vi "AnalogCNTL_MKSorg.vi"() -> ()   [LabVIEW 2015]
uses:
  <userlib>/caLab/Private/Get_PV-1D.vi
panel:
  in  "LocalEpics":u16(ring) items=["LOCAL", "EPCIS"]
  out "APX:HPC100":dbl
  out "APX:HPC01":dbl
  out "Gain":dbl format="%#_6f"
  out "Vin":dbl
  in  "Vref":dbl min=0.0 max=5.0 step=0.01
  in  "ManualAuto":u16(ring) items=["MANUAL", "AUTO"]
  in  "MFC0:Pcell_RQ":dbl
  out "MFC0:Pcell":dbl
  in  "APX:MFC0_Vin":dbl(knob) min=0.0 max=5.0 step=0.001 scale=0.0..5.0
  in  "stop":bool
  # "MFC0"
  # "OPEN"
  # "CLOSE"
  # "MFC"
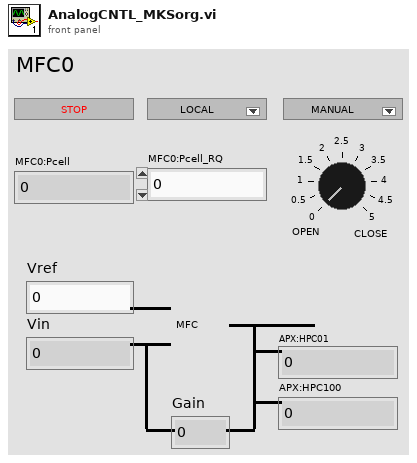
[diagram p1: front panel]
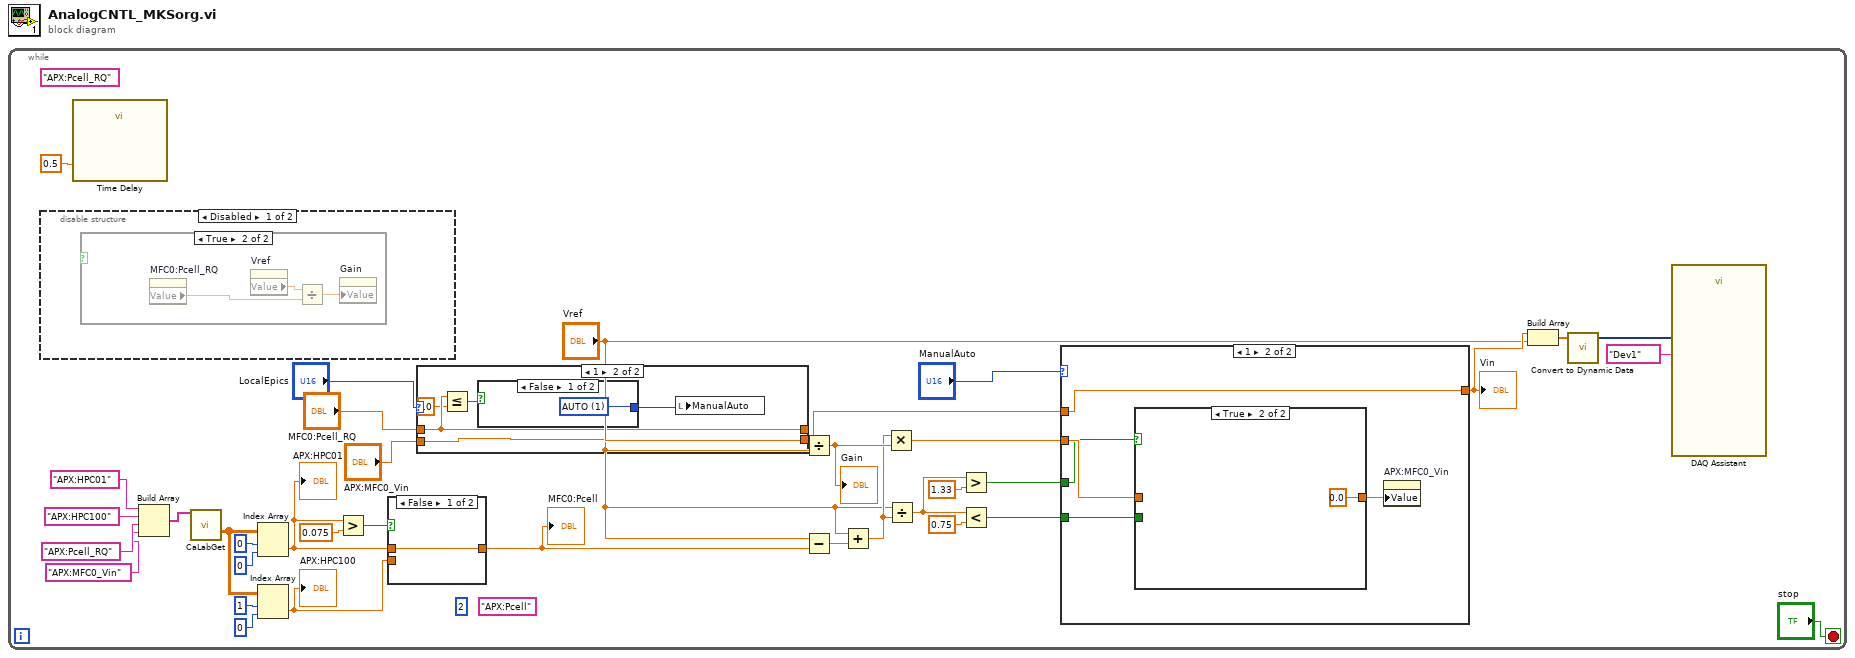
[diagram p0: block diagram]
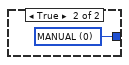
[diagram p4: hidden frame]
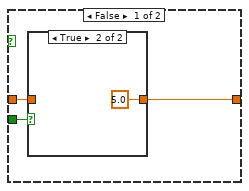
[diagram p8: hidden frame]
diagram:
  n1 = while {
    stop <- "stop" stop-if-true
    (unwired) "APX:Pcell"
    (unwired) "APX:Pcell_RQ"
    (unwired) u16 2 ("y")
    n2 = disable-structure shown="Disabled" {
      frame Disabled {
        n3 = case shown="True" {
          selector: _ -> [_ _]
          frame False {
          }
          frame True {
            n4 = property on="MFC0:Pcell_RQ" class="DigNum (strict)"() -> ("Value"=w49:dbl)  [unwired: 2 in, 2 out]
            n5 = property on="Vref" class="DigNum (strict)"() -> ("Value"=w50:dbl)  [unwired: 2 in, 2 out]
            n6 = Divide(x=w50, y=w49) -> (x/y=w51:dbl)
            n7 = property on="Gain" class="DigNum (strict)"("Value"=w51) -> ()  [unwired: 2 in, 2 out]
          }
        }
      }
      frame Enabled {
      }
    }
    n8 = call "Time Delay"("Delay Time (s)"=0.5) -> ()  [unwired: 10 in, 1 out]
    n9 = Build Array("APX:HPC01", "APX:HPC100", "APX:Pcell_RQ", "APX:MFC0_Vin") -> (w31:string[])
    n10 = call-poly "CaLabGet.vi"("PV Names"=w31) -> ("Value Array (number)"=w27:dbl[][])  [unwired: 8 in, 6 out]
    n11 = Index Array(array=w27, index (row)=0 ("disabled index (col)"), index (col)=0) -> (element=w8:dbl)
    "APX:HPC01" <- w8
    n12 = Index Array(array=w27, index (row)=1 ("disabled index (col)"), index (col)=0) -> (element=w10:dbl)
    "APX:HPC100" <- w10
    n13 = Greater?(x=w8, y=0.075) -> (0:w12:bool)
    n14 = case shown="False" w12 {
      tunnel: w10 -> [_ w39]
      tunnel: [w38 w39] -> w9
      tunnel: w8 -> [w38 _]
      frame False {
      }
      frame True {
      }
    }
    "MFC0:Pcell" <- w9
    n15 = case shown="1" "LocalEpics" {
      tunnel: "MFC0:Pcell_RQ" -> [w41 w45]
      tunnel: [w41 w45] -> w5
      tunnel: [w40 w46] -> w4
      tunnel: "APX:MFC0_Vin" -> [w40 w46]
      frame 0, Default {
      }
      frame 1 {
        n16 = Less Or Equal?(x=w45, y=0.0) -> (x <= y?=w43:bool)
        n17 = case shown="False" w43 {
          tunnel: [w47 w48] -> w42
          frame False {
            w47 = u16 1 items=["MANUAL", "AUTO"] ("ManualAuto")
          }
          frame True {
            w48 = u16 0 items=["MANUAL", "AUTO"] ("ManualAuto")
          }
        }
        n18 = local write "ManualAuto"(w42) -> ()
      }
    }
    n19 = Divide(x="Vref", y=w5) -> (x/y=w16:dbl)
    "Gain" <- w16
    n20 = Subtract(x=w5, y=w9) -> (x-y=w14:dbl)
    n21 = Add(x=w5, y=w14) -> (x+y=w13:dbl)
    n22 = Multiply(x=w13, y=w16) -> (x*y=w34:dbl)
    n23 = Divide(x=w5, y=w13) -> (x/y=w24:dbl)
    n24 = Greater?(x=w24, y=1.33) -> (0:w23:bool)
    n25 = Less?(x=w24, y=0.75) -> (x < y?=w22:bool)
    n26 = case shown="1" "ManualAuto" {
      tunnel: [w52 w57] -> w18
      tunnel: w4 -> [w52 w57]
      tunnel: w34 -> [_ w56]
      tunnel: w23 -> [_ w54]
      tunnel: w22 -> [_ w53]
      frame 0, Default {
      }
      frame 1 {
        n27 = case shown="True" w54 {
          tunnel: w56 -> [w58 _]
          tunnel: [w59 0.0] -> w55
          tunnel: w53 -> [w60 _]
          frame False {
            n28 = case shown="True" w60 {
              tunnel: [w61 5.0] -> w59
              tunnel: w58 -> [w61 _]
              frame False {
              }
              frame True {
              }
            }
          }
          frame True {
          }
        }
        n29 = property on="APX:MFC0_Vin" class="Knob (strict)"("Value"=w55) -> ()  [unwired: 2 in, 2 out]
      }
    }
    "Vin" <- w18
    n30 = Build Array(w18, "Vref") -> (w19:dbl[])
    n31 = call "Convert to Dynamic Data"("Array"=w19) -> ("Dynamic Data Type"=w35:dynamicdata)  [unwired: 3 in]
    n32 = call "DAQ Assistant"("data"=w35, "device name"=tag "Dev1") -> ()  [unwired: 16 in, 2 out]
  }
